vi "Drive Main.vi"() -> ()   [LabVIEW 2013]
uses:
  Robot Global Data.vi
  Controller 1.vi
  <vilib>/Rock Robotics/WPI/RobotDrive/WPI_RobotDriveMecanumDrive_Cartesian.vi
  <vilib>/Rock Robotics/WPI/RobotDrive/WPI_RobotDriveGetSetRefNum.vi
panel:
  in  "Joystick Mult Slow":dbl
  in  "Joystick Mult":dbl
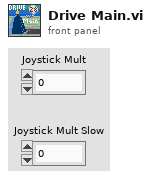
[diagram p1: front panel]
types:
  T1 = cluster{"LS X":dbl, "LS Y":dbl, "Triggers":dbl, "RS X":dbl, "RS Y":dbl}
  T2 = cluster{"A":bool, "B":bool, "X":bool, "Y":bool, "LB":bool, "RB":bool, "Back":bool, "Start":bool, "LS":bool, "RS":bool}
  T3 = typedef "WPI_RobotDriveDevRef.ctl" = cluster{"DevStatus":errorcluster, "Motors[]":T4[], "Square Inputs":bool, "Max Output":dbl, "Isochronous":bool}
  T4 = typedef "WPI_MotorControlDeviceRef.ctl" = cluster{"DeviceStatus":errorcluster, "Type":enum16{"PWM", "CAN"}, "PWM":cluster{"Digital Module":T5, "PWM Channel":T6, "DeadBand":T7}, "CAN":cluster{"Device Number":u8, "Control Mode":T8, "Semaphore":T9, "Max Vout":dbl}, "Invert":bool, "TransformRef":T10, "InvTransformRef":T10}
  T5 = typedef "FPGA_TypedefDigitalModule.ctl" = enum16{"Digital Module 1", "Digital Module 2"}
  T6 = typedef "FPGA_DIOPWMChannel.ctl" = enum8{"PWM 1", "PWM 2", "PWM 3", "PWM 4", "PWM 5", "PWM 6", "PWM 7", "PWM 8", "PWM 9", "PWM 10", "Invalid"}
  T7 = typedef "WPI_PWMDeadband.ctl" = cluster{"Name":string, "maxPositivePwm":i32, "minPositivePwm":i32, "centerPwm":i32, "maxNegativePwm":i32, "minNegativePwm":i32, "angularRange":u16}
  T8 = typedef "WPI_CANJaguar_ControlMode.ctl" = enum8{"Percent VBus", "Current", "Speed", "Position", "Voltage"}
  T9 = typedef "Semaphore RefNum" = refnum<k1>
  T10 = typedef "WPI_PWMTransform_ConPane.ctl" = refnum<vi>
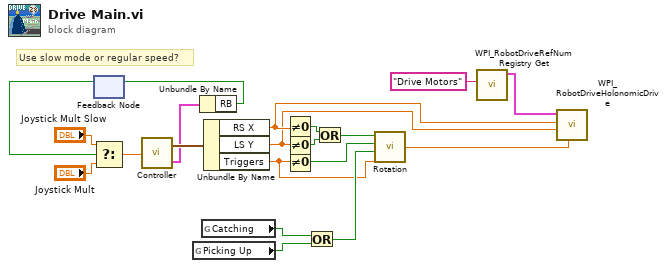
[diagram p0: block diagram]
diagram:
  # "Use slow mode or regular speed?"
  n1 = feedback #1() -> (w5:bool)  [unwired: 1 in]
  n2 = Select(t="Joystick Mult Slow", s=w5, f="Joystick Mult") -> (s? t:f=w8:dbl)
  n3 = call-poly "Controller.vi"("Joystick Multiplier"=w8) -> ("Axes"=w18:T1, "Buttons"=w7:T2)
  n4 = global read "Robot Global Data.vi" "Picking Up"() -> (w1:bool)
  n5 = Unbundle By Name(w7) -> ("RB"=w6:bool)
  n6 = feedback-in #1(w6) -> ()
  n7 = global read "Robot Global Data.vi" "Catching"() -> (w2:bool)
  n8 = Unbundle By Name(w18) -> ("RS X"=w10:dbl, "LS Y"=w9:dbl, "Triggers"=w12:dbl)
  n9 = Not Equal To 0?(x=w10) -> (x != 0?=w14:bool)
  n10 = Not Equal To 0?(x=w9) -> (x != 0?=w17:bool)
  n11 = Not Equal To 0?(x=w12) -> (x != 0?=w15:bool)
  n12 = Or(x=w2, y=w1) -> (x .or. y?=w13:bool)
  n13 = Or(x=w14, y=w17) -> (x .or. y?=w16:bool)
  n14 = call "Rotation.vi"("Uncorrected Speed"=w12, "Tracking Ball"=w13, "Rotating Manually"=w15, "Moving Laterally"=w16) -> ("Output Speed"=w11:dbl)
  n15 = call <vilib>:"WPI_RobotDriveRefNum Registry Get.vi"("refnum name"="Drive Motors") -> ("RobotDriveDevRef"=w20:T3)  [unwired: 1 in, 9 out]
  n16 = call-poly <vilib>:"WPI_RobotDriveHolonomicDrive.vi"("Rotation"=w11, "Y"=w9, "X"=w10, "RobotDriveDevRef"=w20) -> ()  [unwired: 5 in, 3 out]
